vi "SaveStop.vi"(11 "TDMSFile":refnum<k34>) -> ()   [LabVIEW 2019]
panel:
  # "This Vi closes  the TDMS files in which the setting and data is saved."
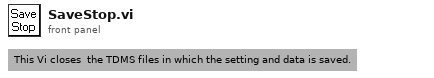
[diagram p1: front panel]
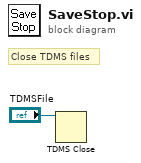
[diagram p0: block diagram]
diagram:
  # "Close TDMS files"
  n1 = TDMS Close(11:"TDMSFile") -> ()  [unwired: 1 in, 2 out]
